vi "Create CSS Variables.vi"(11 "light":T1) -> (3 "CSS":string)   [LabVIEW 2021, in "TSC Material Theme.lvlib" / "Material-Scheme.lvclass"]
doc: "for when new browser plugins get implemented, apply variables for CSS from the color scheme\n\n<b>Code Developed By:</b>\nTechnology Service Corporation\nwww.tsc.com/atcs\n\nDeveloper:\nDaniel Coons"
uses:
  Material-Scheme.lvclass
  _Material Theme SubVIs/material json scheme.ctl
  Material-Scheme.lvclass/Material-Scheme.ctl
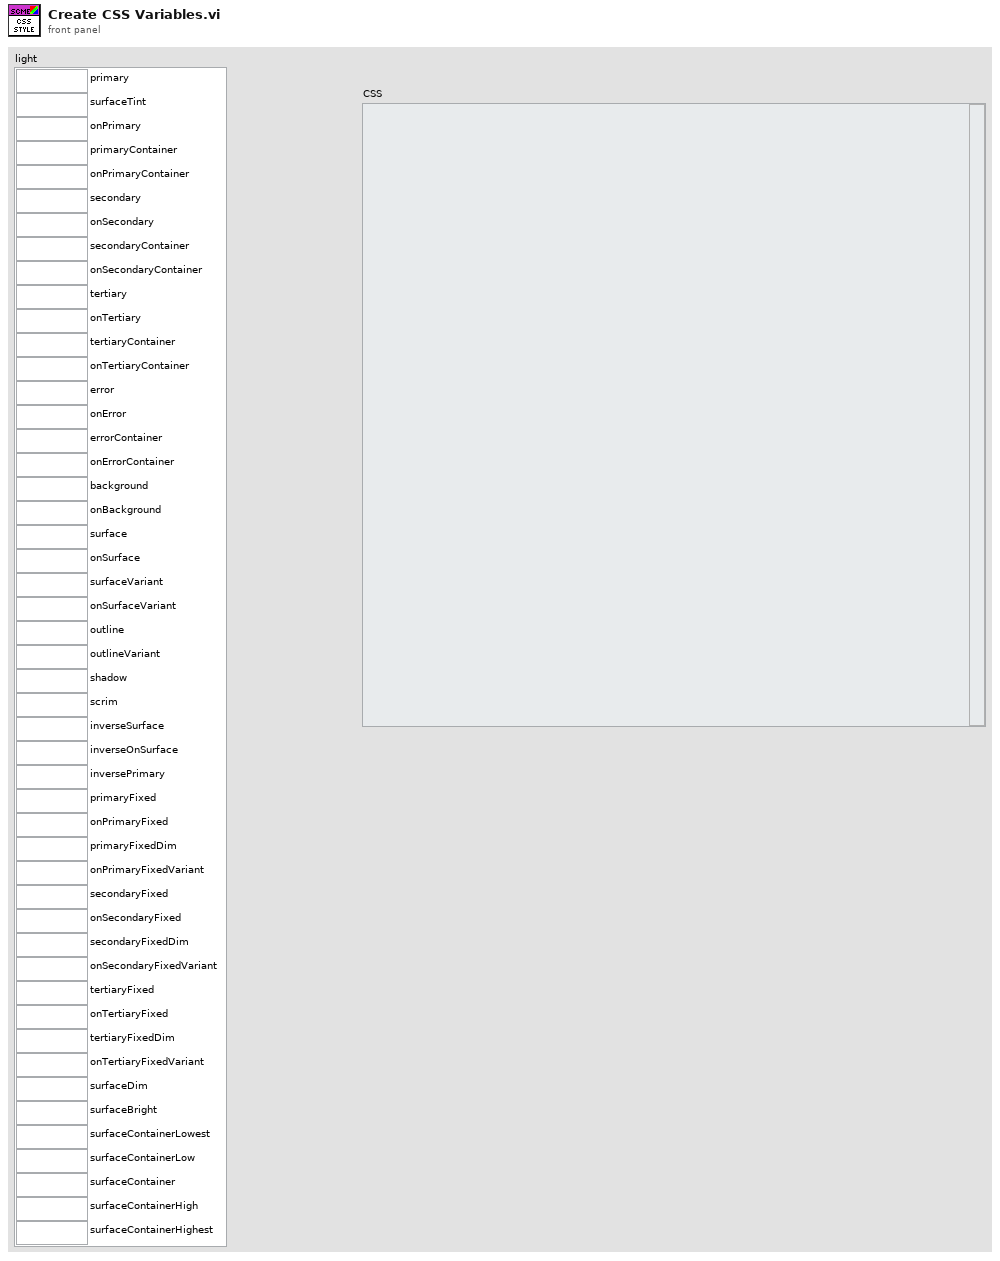
[diagram p1: front panel]
types:
  T1 = typedef "material json scheme.ctl" = cluster{"primary":string, "surfaceTint":string, "onPrimary":string, "primaryContainer":string, "onPrimaryContainer":string, "secondary":string, "onSecondary":string, "secondaryContainer":string, "onSecondaryContainer":string, "tertiary":string, "onTertiary":string, "tertiaryContainer":string, "onTertiaryContainer":string, "error":string, "onError":string, "errorContainer":string, "onErrorContainer":string, "background":string, "onBackground":string, "surface":string, "onSurface":string, "surfaceVariant":string, "onSurfaceVariant":string, "outline":string, "outlineVariant":string, "shadow":string, "scrim":string, "inverseSurface":string, "inverseOnSurface":string, "inversePrimary":string, "primaryFixed":string, "onPrimaryFixed":string, "primaryFixedDim":string, "onPrimaryFixedVariant":string, "secondaryFixed":string, "onSecondaryFixed":string, "secondaryFixedDim":string, "onSecondaryFixedVariant":string, "tertiaryFixed":string, "onTertiaryFixed":string, "tertiaryFixedDim":string, "onTertiaryFixedVariant":string, "surfaceDim":string, "surfaceBright":string, "surfaceContainerLowest":string, "surfaceContainerLow":string, "surfaceContainer":string, "surfaceContainerHigh":string, "surfaceContainerHighest":string}
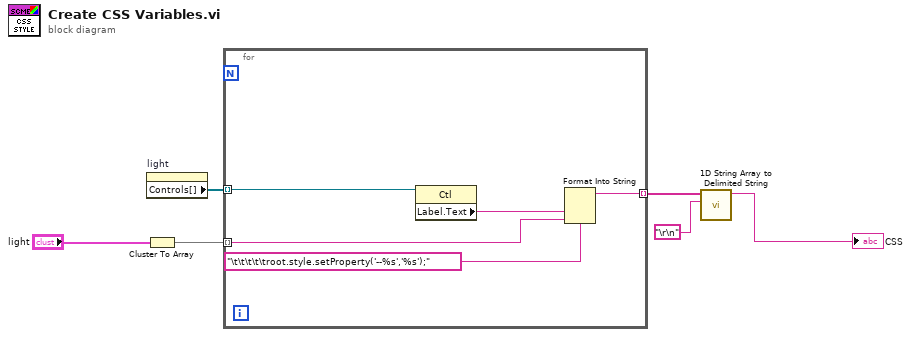
[diagram p0: block diagram]
diagram:
  n1 = property on="light" class="Clust (strict)"() -> ("Controls[]"=w4:refnum<vi>[])  [unwired: 2 in, 2 out]
  n2 = Cluster To Array(cluster="light") -> (array=w6:string[])
  n3 = for {
    tunnel: w6 -> [w8] mode=indexing
    tunnel: w4 -> [w11] mode=indexing
    tunnel: [w7] -> w3 mode=indexing
    n4 = property class="Ctl"(reference=w11) -> ("Label.Text"=w9:string)  [unwired: 1 in, 2 out]
    n5 = Format Into String(format string="\t\t\t\t\troot.style.setProperty('--%s','%s');", w9, w8) -> (resulting string=w7:string)  [unwired: 2 in, 1 out]
  }
  n6 = call <vilib>:"1D String Array to Delimited String.vi"("delimiter"="\r\n", "string array"=w3) -> ("delimited string"=→"CSS":string)  [unwired: 9 in]
